vi "temp.array.vi"(11 "dbg.state":T2={"state"=enum."Wait", "arr"=[0, 0, 0, 0], "index"=0, "TLAST"=FALSE, "TDATA"=0}) -> ()   [LabVIEW 2020]
uses:
  submodules/Market.Data.Bats.Parser/fpga/poc.ip.debug.states.ctl
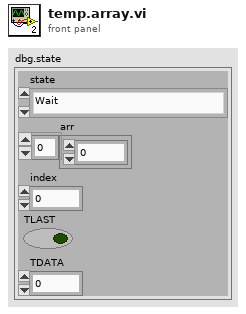
[diagram p1: front panel]
types:
  T1 = typedef "poc.ip.debug.states.ctl" = enum16{"Wait", "Write.Data"}
  T2 = cluster{"state":T1, "arr":u64[], "index":u8, "TLAST":bool, "TDATA":u64}
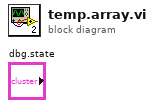
[diagram p0: block diagram]
diagram:
